vi "Close DB Reference.vi"(8 "error in (no error)":errorcluster, 11 "MySQL in":refnum<class "MySQL.lvclass">) -> (0 "error out":errorcluster, 3 "MySQL out":refnum<class "MySQL.lvclass">)   [LabVIEW 2016, in "Database.lvlib" / "MySQL.lvclass"]
uses:
  MySQL.lvclass
  MySQL.lvclass/MySQL.ctl
  <vilib>/addons/database/Connection.llb/Conn ObjectReference.ctl
  <vilib>/addons/database/NI_Database_API.lvlib
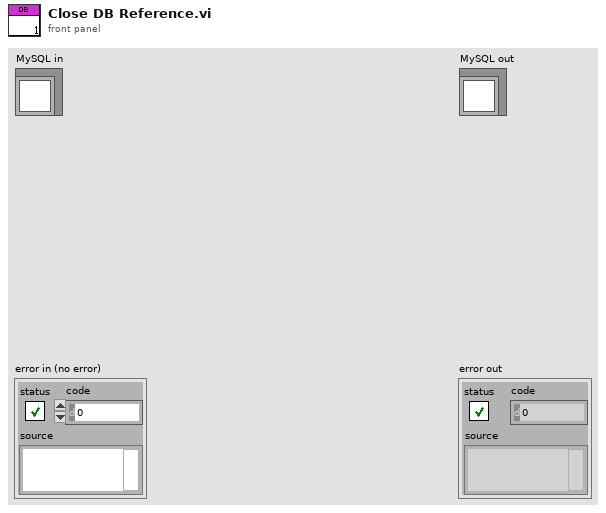
[diagram p1: front panel]
types:
  T1 = typedef "NI_Database_API.lvlib/Conn ObjectReference.ctl" = refnum<k1>
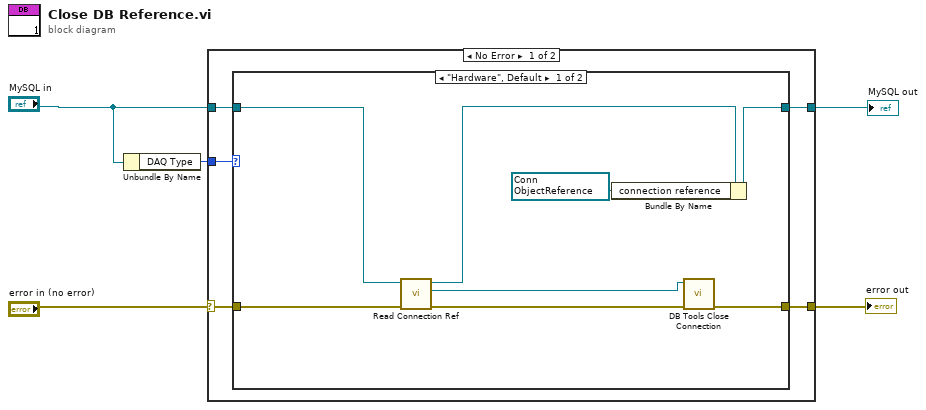
[diagram p0: block diagram]
diagram:
  n1 = Unbundle By Name("MySQL in") -> ("DAQ Type"=w5:enum16{"Hardware", "Simulation"})
  n2 = case shown="No Error" "error in (no error)" {
    selector: "error in (no error)" -> [w10 w21]
    tunnel: [w9 w22] -> w2
    tunnel: [w8 w21] -> w1
    tunnel: "MySQL in" -> [w7 w22]
    tunnel: w5 -> [w6 _]
    frame No Error {
      n3 = case shown="\"Hardware\", Default" w6 {
        tunnel: w10 -> [w11 w19]
        tunnel: [w18 w20] -> w9
        tunnel: [w17 w19] -> w8
        tunnel: w7 -> [w16 w20]
        frame "Hardware", Default {
          w13 = T1 refnum items=["Connection"] ("connection reference")
          n4 = call-dynamic "Read Connection Ref.vi"("error in (no error)"=w11, "MySQL in"=w16) -> ("error out"=w15:errorcluster, "connection reference"=w14:T1, "MySQL out"=w12:refnum<class "MySQL.lvclass">)  [unwired: 7 in]
          n5 = Bundle By Name(cluster=w12, "connection reference"=w13) -> (w18:refnum<class "MySQL.lvclass">)
          n6 = call <vilib>:"DB Tools Close Connection.vi"("error in (no error)"=w15, "connection reference"=w14) -> ("error out"=w17:errorcluster)  [unwired: 5 in]
        }
        frame "Simulation" {
        }
      }
    }
    frame Error {
    }
  }
  "error out" <- w1
  "MySQL out" <- w2
